vi "Jens.vi"(9 "REPL":string, 10 "Send":string) -> ()   [LabVIEW 2020]
uses:
  <vilib>/Instr/_visa.llb/VISA Configure Serial Port (Instr).vi
panel:
  in  "Status":bool
  out "Cover":bool
  in  "Script":string
  in  "Buffer":string
  in  "Disconnect":bool
  in  "Help":bool
  in  "Connect":bool
  in  "Stop Button":bool
  in  "Port":refnum<visa-resource-name>
  out "Running Script":bool
  in  "Abort":bool
  in  "xPort":string
  out "Status":T1 {"Accel" scale=-1000.0..1000.0; "Position" scale=-100.0..360.0; "Gyro" scale=-1000.0..1000.0}
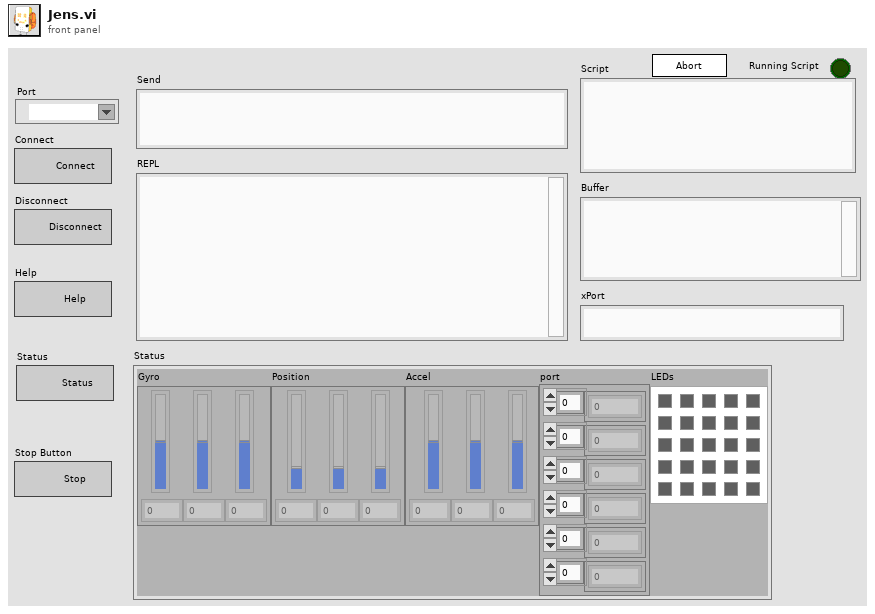
[diagram p1: front panel]
types:
  T1 = cluster{"Gyro":i32[], "Position":i32[], "Accel":i32[], "port":cluster{"A":i32[], "B":i32[], "C":i32[], "D":i32[], "E":i32[], "F":i32[]}, "LEDs":u32[][]}
  T2 = enum32{"Invalid", "Standard", "Closed", "Hidden", "Minimized", "Maximized"}
  T3 = typedef "eventvkey.ctl" = enum16{"ASCII", "Enter", "Return", "Shift", "Ctrl", "Alt", "Cmd", "Opt", "Caps", "NumLock", "Clear", "Break", "Up", "Down", "Left", "Right", "Insert", "Delete", "Home", "End", "PageUp", "PageDown", "Escape", "Help", "Pause", "ScrollLock", "F1", "F2", "F3", "F4", "F5", "F6", "F7", "F8", "F9", "F10", "F11", "F12", "F13", "F14", "F15", "F16", "F17", "F18", "F19", "F20", "F21", "F22", "F23", "F24", "Play", "VolumeUp", "VolumeDown", "Mute", "Two Byte Char"}
  T4 = cluster{"Shift":bool, "Ctrl":bool, "Alt":bool, "Cmd":bool, "Opt":bool}
  T5 = cluster{"Char":i16, "VKey":T3, "PlatMods":cluster{"Shift":bool, "Ctrl":bool, "Alt":bool, "Cmd":bool, "Opt":bool}}
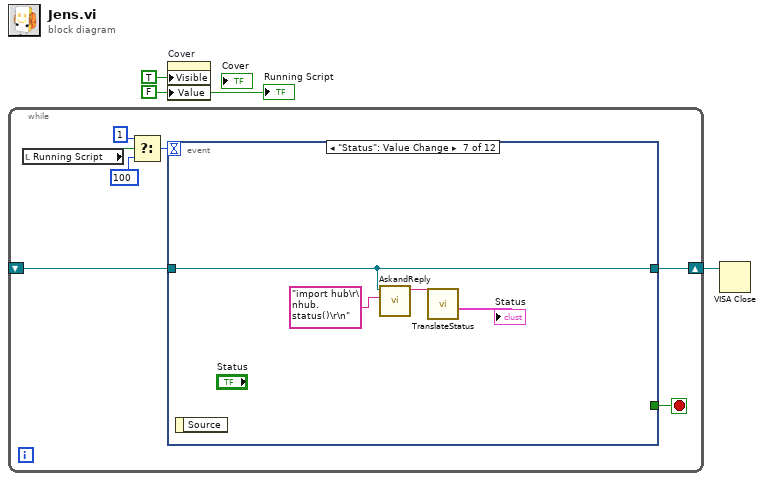
[diagram p0: block diagram]
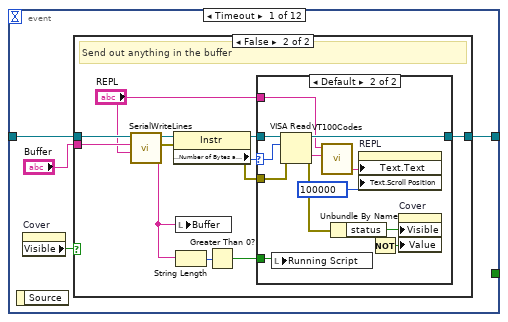
[diagram p2: hidden frame]
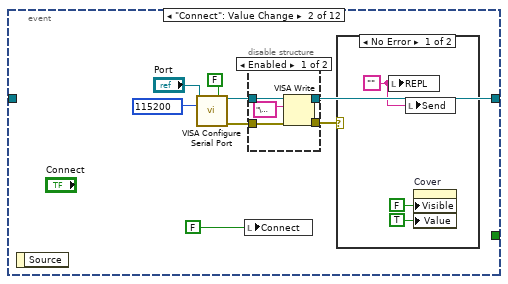
[diagram p5: hidden frame]
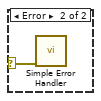
[diagram p7: hidden frame]
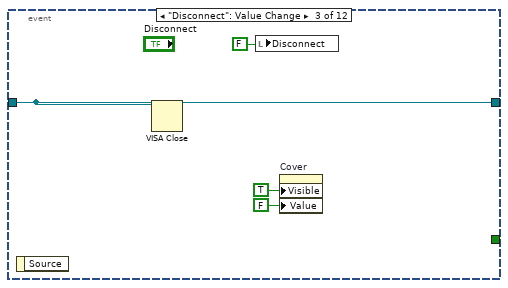
[diagram p8: hidden frame]
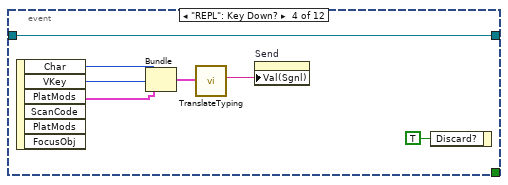
[diagram p9: hidden frame]
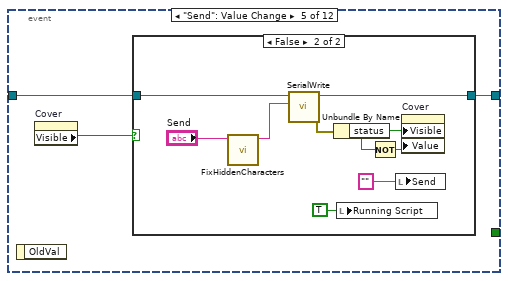
[diagram p10: hidden frame]
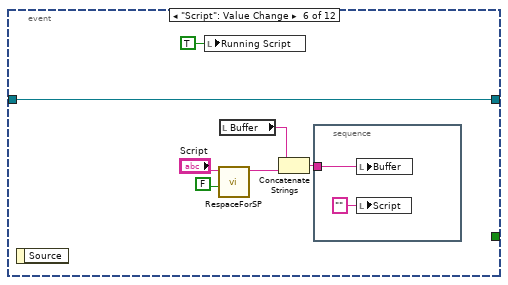
[diagram p12: hidden frame]
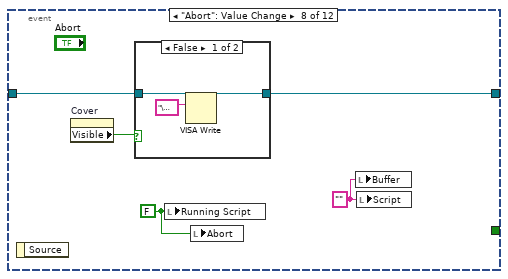
[diagram p13: hidden frame]
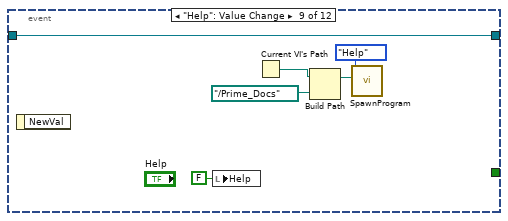
[diagram p15: hidden frame]
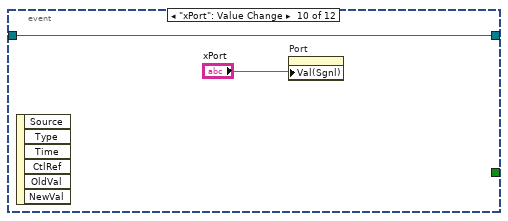
[diagram p16: hidden frame]
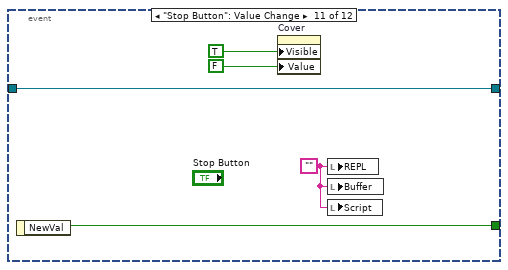
[diagram p17: hidden frame]
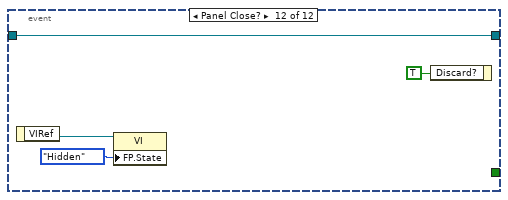
[diagram p18: hidden frame]
diagram:
  w1 = FALSE ("Cover")
  n1 = while {
    shift-right: [w9] -> w2
    shift-left: _ -> [w8]
    stop <- w10 stop-if-true
    n2 = local read "Running Script"() -> (w4:bool)
    n3 = Select(t=1, s=w4, f=100) -> (s? t:f=w5:i32)
    n4 = event shown="[6] \"Status\": Value Change" {
      selector: _ -> [_ _ _ _ _ _ _ _ _ _ _ _]
      dyn-events: _ -> [_ _ _ _ _ _ _ _ _ _ _ _]
      timeout: w5 -> [_ _ _ _ _ _ _ _ _ _ _ _]
      tunnel: [_ _ _ _ _ _ _ _ _ _ w116 _] -> w10
      tunnel: [w14 w44 w62 w69 w71 w87 w95 w99 w110 w112 w117 w121] -> w9
      tunnel: w8 -> [w13 _ w62 w69 w72 w87 w95 w98 w110 w112 w117 w121]
      event Timeout {
        n5 = event-data() -> ()  [unwired: 1 in, 1 out]
        n6 = property on="Cover" class="Bool (strict)"() -> ("Visible"=w12:bool)  [unwired: 2 in, 2 out]
        n7 = case shown="False" w12 {
          tunnel: [w15 w26] -> w14
          tunnel: w13 -> [w15 w25]
          tunnel: "Buffer" -> [_ w24]
          frame True {
          }
          frame False {
            # "Send out anything in the buffer"
            n8 = call "SerialWriteLines.vi"("REPL"="REPL", "Send"=w24, "VISA Refnum in"=w25) -> ("error out"=w21:errorcluster, "Rest"=w18:string, "VISA Refnum out"=w23:refnum<visa-resource-name>)  [unwired: 6 in]
            n9 = property class="Instr"(reference=w23, error in=w21) -> (error out=w20:errorcluster, "Serial Settings:Number of Bytes at Serial Port"=w22:u32)  [unwired: 1 out]
            n10 = local write "Buffer"(w18) -> ()
            n11 = String Length(string=w18) -> (length=w19:i32)
            n12 = Greater Than 0?(x=w19) -> (x > 0?=w17:bool)
            n13 = case shown="Default" w22 {
              selector: w22 -> [_ w35]
              tunnel: [w27 w39] -> w26
              tunnel: w23 -> [w27 w38]
              tunnel: w20 -> [_ w33]
              tunnel: w17 -> [_ w31]
              tunnel: "REPL" -> [_ w30]
              frame 0 {
              }
              frame Default {
                n14 = local write "Running Script"(w31) -> ()
                n15 = VISA Read(VISA resource name=w38, byte count=w35, error in (no error)=w33) -> (VISA resource name out=w39:refnum<visa-resource-name>, read buffer=w36:string, error out=w32:errorcluster)  [unwired: 1 out]
                n16 = call "VT100Codes.vi"("read buffer"=w36, "Console In"=w30) -> ("Console Out"=w34:string)  [unwired: 9 in]
                n17 = Unbundle By Name(w32) -> ("status"=w28:bool)
                n18 = property on="REPL" class="Str"("Text.Text"=w34, "Text.Scroll Position"=u32 100000 ("Text.Selection:Start")) -> ()  [unwired: 2 in, 2 out]
                n19 = Not(x=w28) -> (.not. x?=w29:bool)
                n20 = property on="Cover" class="Bool (strict)"("Visible"=w28, "Value"=w29) -> ()  [unwired: 2 in, 2 out]
              }
            }
          }
        }
      }
      event "Connect": Value Change {
        n21 = event-data() -> ()  [unwired: 1 in, 1 out]
        n22 = call-poly "VISA Configure Serial Port"("VISA resource name"="Port", "Enable Termination\nChar (T)"=FALSE ("Enable Termination\nChar (T)"), "baud rate (9600)"=u32 115200) -> ("VISA resource name out"=w45:refnum<visa-resource-name>, "error out"=w43:errorcluster)  [unwired: 11 in]
        n23 = local write "Connect"(FALSE ("Help")) -> ()
        n24 = disable-structure shown="Enabled" {
          disable-tunnel: w45 -> [w52 w54]
          disable-tunnel: [w51 w54] -> w44
          disable-tunnel: w43 -> [w50 w53]
          disable-tunnel: [w49 w53] -> w42
          frame Enabled {
            n25 = VISA Write(VISA resource name=w52, write buffer="\u0003", error in (no error)=w50) -> (VISA resource name out=w51:refnum<visa-resource-name>, error out=w49:errorcluster)  [unwired: 1 out]
          }
          frame Disabled {
          }
        }
        n26 = case shown="No Error" w42 {
          selector: w42 -> [_ w58]
          frame No Error {
            w57 = ""
            n27 = local write "REPL"(w57) -> ()
            n28 = local write "Send"(w57) -> ()
            n29 = property on="Cover" class="Bool (strict)"("Visible"=FALSE, "Value"=TRUE ("Cover")) -> ()  [unwired: 2 in, 2 out]
          }
          frame Error {
            n30 = call <vilib>:"Simple Error Handler.vi"("error in (no error)"=w58) -> ()  [unwired: 4 in, 5 out]
          }
        }
      }
      event "Disconnect": Value Change {
        n31 = event-data() -> ()  [unwired: 1 in, 1 out]
        n32 = VISA Close(VISA resource name=w62) -> ()  [unwired: 1 in, 1 out]
        n33 = local write "Disconnect"(FALSE ("Help")) -> ()
        n34 = property on="Cover" class="Bool (strict)"("Visible"=TRUE, "Value"=FALSE ("Cover")) -> ()  [unwired: 2 in, 2 out]
      }
      event "REPL": Key Down? {
        n35 = event-data() -> ("Char"=w65:i16, "VKey"=w66:T3, "PlatMods"=w67:T4)  [unwired: 1 in, 3 out]
        n36 = Bundle("Char"=w65, "VKey"=w66, "PlatMods"=w67) -> (w68:T5)  [unwired: 1 in]
        n37 = call "TranslateTyping.vi"("Cluster"=w68) -> ("key"=w64:string)  [unwired: 10 in]
        n38 = property on="Send" class="Str"("Val(Sgnl)"=w64) -> ()  [unwired: 2 in, 2 out]
        n39 = event-data("Discard?"=TRUE) -> ()  [unwired: 1 in, 1 out]
      }
      event "Send": Value Change {
        n40 = event-data() -> ()  [unwired: 1 in, 1 out]
        n41 = property on="Cover" class="Bool (strict)"() -> ("Visible"=w70:bool)  [unwired: 2 in, 2 out]
        n42 = case shown="False" w70 {
          tunnel: w72 -> [w73 w82]
          tunnel: [w73 w81] -> w71
          frame True {
          }
          frame False {
            n43 = call "FixHiddenCharacters.vi"("String in"="Send") -> ("String out"=w77:string)  [unwired: 10 in]
            n44 = call "SerialWrite.vi"("Text"=w77, "VISA Refnum in"=w82) -> ("error out"=w74:errorcluster, "VISA Refnum out"=w81:refnum<visa-resource-name>)  [unwired: 8 in]
            n45 = Unbundle By Name(w74) -> ("status"=w75:bool)
            n46 = local write "Running Script"(TRUE ("Running Script")) -> ()
            n47 = Not(x=w75) -> (.not. x?=w76:bool)
            n48 = local write "Send"("" ("Write text")) -> ()
            n49 = property on="Cover" class="Bool (strict)"("Visible"=w75, "Value"=w76) -> ()  [unwired: 2 in, 2 out]
          }
        }
      }
      event "Script": Value Change {
        n50 = event-data() -> ()  [unwired: 1 in, 1 out]
        n51 = local write "Running Script"(TRUE ("Visible")) -> ()
        n52 = call "RespaceForSP.vi"("Keep spaces?"=FALSE, "Code"="Script") -> ("Cleaned for SPIKE"=w84:string)  [unwired: 9 in]
        n53 = local read "Buffer"() -> (w85:string)
        n54 = Concatenate Strings(w85, w84) -> (w83:string)
        n55 = stacked-sequence {
          tunnel: w83 -> [w91]
          frame #0 {
            n56 = local write "Buffer"(w91) -> ()
            n57 = local write "Script"("" ("Script")) -> ()
          }
        }
      }
      event "Status": Value Change {
        n58 = event-data() -> ()  [unwired: 1 in, 1 out]
        n59 = call "AskandReply.vi"("Send"="import hub\r\nhub.status()\r\n", "VISA Refnum in"=w95) -> ("Reply"=w93:string)  [unwired: 9 in]
        n60 = call "TranslateStatus.vi"("Reply"=w93) -> ("Status"=→"Status":T1)  [unwired: 9 in, 1 out]
      }
      event "Abort": Value Change {
        w100 = "" ("Script")
        w97 = FALSE ("Visible")
        n61 = event-data() -> ()  [unwired: 1 in, 1 out]
        n62 = property on="Cover" class="Bool (strict)"() -> ("Visible"=w96:bool)  [unwired: 2 in, 2 out]
        n63 = case shown="False" w96 {
          tunnel: [w102 w104] -> w99
          tunnel: w98 -> [w101 w104]
          frame False {
            n64 = VISA Write(VISA resource name=w101, write buffer="\u0003") -> (VISA resource name out=w102:refnum<visa-resource-name>)  [unwired: 1 in, 2 out]
          }
          frame True {
          }
        }
        n65 = local write "Running Script"(w97) -> ()
        n66 = local write "Abort"(w97) -> ()
        n67 = local write "Buffer"(w100) -> ()
        n68 = local write "Script"(w100) -> ()
      }
      event "Help": Value Change {
        n69 = event-data() -> ()  [unwired: 1 in, 1 out]
        n70 = local write "Help"(FALSE ("Help")) -> ()
        n71 = Current VI's Path() -> (path=w108:path)
        n72 = Build Path(base path=w108, name or relative path=path "../Prime_Docs") -> (appended path=w106:path)
        n73 = call "SpawnProgram.vi"("Server"=w106, "Dialog"=enum16{"Help", "Files"}."Help") -> ()  [unwired: 10 in]
      }
      event "xPort": Value Change {
        n74 = event-data() -> ()  [unwired: 1 in, 6 out]
        n75 = property on="Port" class="VISAName"("Val(Sgnl)"="xPort") -> ()  [unwired: 2 in, 2 out]
      }
      event "Stop Button": Value Change {
        w113 = ""
        n76 = event-data() -> ("NewVal"=w116:bool)  [unwired: 1 in]
        n77 = property on="Cover" class="Bool (strict)"("Visible"=TRUE, "Value"=FALSE ("Cover")) -> ()  [unwired: 2 in, 2 out]
        n78 = local write "REPL"(w113) -> ()
        n79 = local write "Buffer"(w113) -> ()
        n80 = local write "Script"(w113) -> ()
      }
      event Panel Close? {
        n81 = event-data() -> ("VIRef"=w119:refnum<vi>)  [unwired: 1 in]
        n82 = property class="VI"(reference=w119, "FP.State"=T2."Hidden" ("Front Panel Window:State")) -> ()  [unwired: 1 in, 2 out]
        n83 = event-data("Discard?"=TRUE) -> ()  [unwired: 1 in, 1 out]
      }
    }
  }
  n84 = property on="Cover" class="Bool (strict)"("Visible"=TRUE, "Value"=w1) -> ()  [unwired: 2 in, 2 out]
  n85 = VISA Close(VISA resource name=w2) -> ()  [unwired: 1 in, 1 out]
  "Running Script" <- w1
